vi "read_config_settings.vi"() -> ()   [LabVIEW 2011]
doc: "Illustrates how to read a configuration settings file.\n\nInstructions:\nRun Write Configuration Settings File.vi, located in the file\\config.llb. Then run this VI and select the appropriate configuration settings file to load."
uses:
  <vilib>/Utility/config.llb/Read Key (Boolean).vi
  <vilib>/Utility/config.llb/Read Key (Double).vi
  <vilib>/Utility/config.llb/Read Key (Path).vi
  <vilib>/Utility/config.llb/Read Key (String).vi
  <vilib>/Utility/config.llb/NI_LVConfig.lvlib
panel:
  out "Path Value":path
  out "Numeric":dbl format="%0.2f"
  out "Boolean":bool
  out "String 2":string
  out "String 1":string
  # "Instructions:\nRun Write Configuration Settings File.vi, located in the file\\config.llb, first.\nThen run this VI and select the appropriate configuration settings file to load."
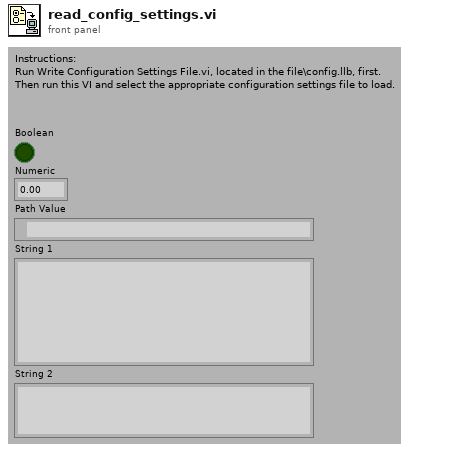
[diagram p1: front panel]
types:
  T1 = typedef "NI_LVConfig.lvlib/Config Data RefNum.ctl" = refnum<k1>
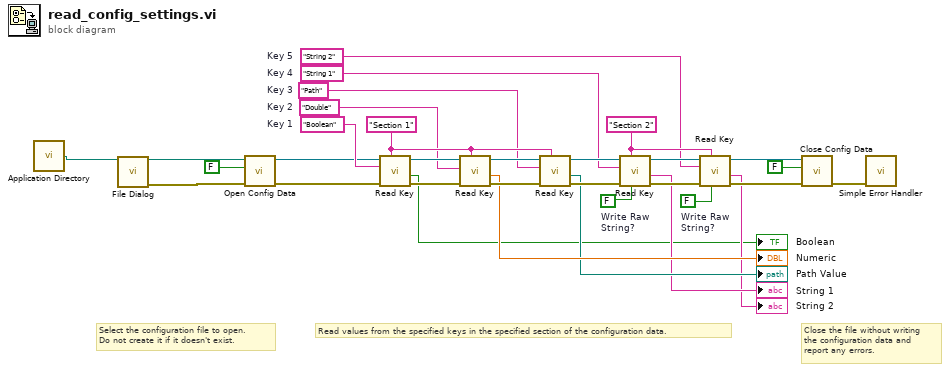
[diagram p0: block diagram]
diagram:
  w6 = FALSE  # Write Raw String?
  w7 = FALSE  # Write Raw String?
  w16 = "String 2"  # Key 5
  w17 = "String 1"  # Key 4
  w18 = "Path"  # Key 3
  w19 = "Double"  # Key 2
  w20 = "Boolean"  # Key 1
  w21 = "Section 2" ("section")
  w22 = "Section 1" ("section")
  # "Close the file without writing\nthe configuration data and\nreport any errors."
  # "Read values from the specified keys in the specified section of the configuration data."
  # "Select the configuration file to open.\nDo not create it if it doesn't exist."
  n1 = call <vilib>:"Application Directory.vi"() -> ("Application Directory"=w3:path)
  n2 = call "File Dialog"("start path"=w3) -> ("selected path"=w2:path, "error out"=w1:errorcluster)  [unwired: 11 in, 2 out]
  n3 = call <vilib>:"Open Config Data.vi"("error in (no error)"=w1, "create file if necessary (T)"=FALSE ("create file if necessary? (T)"), "configuration file path"=w2) -> ("error out"=w14:errorcluster, "refnum"=w13:T1)  [unwired: 6 in, 1 out]
  n4 = call-poly <vilib>:"Read Key.vi"("section"=w22, "error in (no error)"=w14, "key"=w20, "refnum"=w13) -> ("error out"=w32:errorcluster, "value"=→"Boolean":bool, "refnum out"=w30:T1)  [unwired: 1 in, 4 out]
  n5 = call-poly <vilib>:"Read Key.vi"("section"=w22, "error in (no error)"=w32, "key"=w19, "refnum"=w30) -> ("error out"=w27:errorcluster, "value"=→"Numeric":dbl, "refnum out"=w28:T1)  [unwired: 1 in, 4 out]
  n6 = call-poly <vilib>:"Read Key.vi"("section"=w22, "error in (no error)"=w27, "key"=w18, "refnum"=w28) -> ("error out"=w31:errorcluster, "value"=→"Path Value":path, "refnum out"=w29:T1)  [unwired: 1 in, 4 out]
  n7 = call-poly <vilib>:"Read Key.vi"("read raw string? (F)"=w6, "section"=w21, "error in (no error)"=w31, "key"=w17, "refnum"=w29) -> ("error out"=w24:errorcluster, "value"=→"String 1":string, "refnum out"=w23:T1)  [unwired: 1 in, 3 out]
  n8 = call-poly <vilib>:"Read Key.vi"("read raw string? (F)"=w7, "section"=w21, "error in (no error)"=w24, "key"=w16, "refnum"=w23) -> ("error out"=w26:errorcluster, "value"=→"String 2":string, "refnum out"=w25:T1)  [unwired: 1 in, 3 out]
  n9 = call <vilib>:"Close Config Data.vi"("error in (no error)"=w26, "write file if changed (T)"=FALSE ("write configuration file? (T)"), "refnum"=w25) -> ("error out"=w15:errorcluster)  [unwired: 8 out]
  n10 = call <vilib>:"Simple Error Handler.vi"("error in (no error)"=w15) -> ()  [unwired: 1 in, 8 out]
